vi "GetStringPropertyValueInClusterArray.vi"(0 "Array In":cluster{".NET Refnum":refnum<k24>}[](array[cluster])) -> (1 "Array Out":cluster{".NET Refnum":refnum<k24>}[](array[cluster]), 2 "String Value Property":string, 3 "error out":errorcluster)   [LabVIEW 2010]
uses:
  \\camila\f$/Tests/LVBuildValidation/10.0/Automated/FlexLVAdapter30/Refnums/DotNetRefnum/LabviewDNTest.dll
  LabviewDNTest.dll
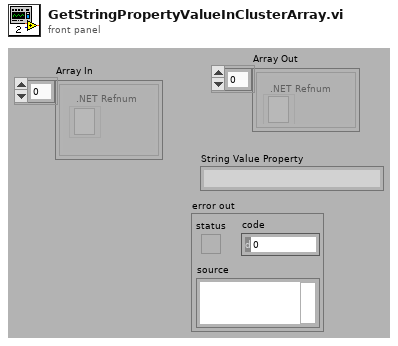
[diagram p1: front panel]
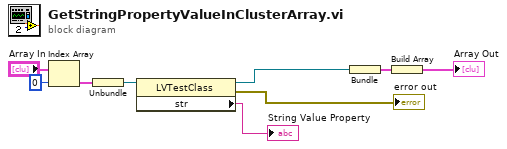
[diagram p0: block diagram]
diagram:
  n1 = Index Array(array="Array In", index=0) -> (element=w7:cluster{".NET Refnum":refnum<k24>})
  n2 = Unbundle(w7) -> (".NET Refnum"=w4:refnum<k24>)
  n3 = property class="LVTestClass"(reference=w4) -> (reference out=w3:refnum<k24>, error out=→"error out":errorcluster, "str"=→"String Value Property":string)  [unwired: 1 in]
  n4 = Bundle(".NET Refnum"=w3) -> (w6:cluster{".NET Refnum":refnum<k24>})  [unwired: 1 in]
  n5 = Build Array(w6) -> (→"Array Out":cluster{".NET Refnum":refnum<k24>}[])
